vi "WriteToDisk.vi"(8 "error in (no error)":errorcluster, 11 "Electrophysiology.lvclass":refnum<class "Electrophysiology.lvclass">) -> (0 "error out":errorcluster, 2 "Writing Backlog":i32, 3 "Electrophysiology.lvclass out":refnum<class "Electrophysiology.lvclass">)   [LabVIEW 2014, in "Electrophysiology.lvclass"]
uses:
  Electrophysiology.lvclass
  Electrophysiology.lvclass/Electrophysiology.ctl
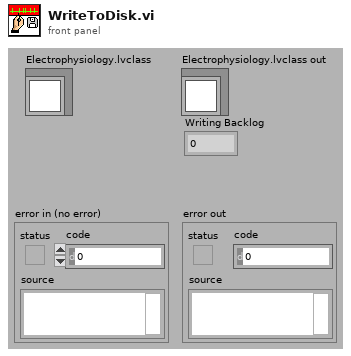
[diagram p1: front panel]
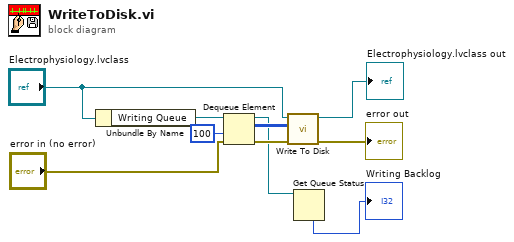
[diagram p0: block diagram]
diagram:
  n1 = Unbundle By Name("Electrophysiology.lvclass") -> ("Writing Queue"=w10:refnum<queue>)
  n2 = Dequeue Element(queue=w10, timeout in ms (-1)=100, error in (no error)="error in (no error)") -> (queue out=w2:refnum<queue>, element=w7:i32[][], error out=w8:errorcluster)  [unwired: 1 out]
  n3 = call-dynamic "Write To Disk.vi"("error in (no error)"=w8, "element"=w7, "AcquireTraces in"="Electrophysiology.lvclass") -> ("error out"=→"error out":errorcluster, "AcquireTraces out"=→"Electrophysiology.lvclass out":refnum<class "Electrophysiology.lvclass">)  [unwired: 7 in]
  n4 = Get Queue Status(queue=w2) -> (# elements in queue=→"Writing Backlog":i32)  [unwired: 2 in, 7 out]
